vi "CreateQbusListners.vi"(11 "ConnInfo":T1) -> (0 "error out":errorcluster, 3 "Qbus out":refnum<class "Qbus.lvclass">)   [LabVIEW 2017]
uses:
  <vilib>/addons/Qbus/Qbus.lvclass
  <vilib>/addons/InsightCM/Devices/Shared/Common/ServerComm/ServerComm.lvlib
  <vilib>/addons/TimerProcess/TimerProcess.lvlib
  <vilib>/addons/InsightCM/Devices/Shared/Common/DataFlow/test/SpeedBenchmark/Loop1/Loop1.lvlib
  <vilib>/addons/InsightCM/Devices/Shared/Common/DataFlow/test/SpeedBenchmark/Loop2/Loop2.lvlib
  <vilib>/addons/InsightCM/Devices/Shared/Common/DataFlow/test/SpeedBenchmark/Loop3/Loop3.lvlib
  <vilib>/addons/InsightCM/Devices/Shared/Common/DataFlow/test/SpeedBenchmark/Loop4/Loop4.lvlib
  <vilib>/addons/InsightCM/Devices/Shared/Common/DataFlow/test/SpeedBenchmark/Loop5/Loop5.lvlib
  <vilib>/addons/InsightCM/Devices/Shared/Common/DataFlow/test/SpeedBenchmark/Loop6/Loop6.lvlib
  <vilib>/addons/InsightCM/Devices/Shared/Common/DataFlow/test/SpeedBenchmark/Loop7/Loop7.lvlib
  <vilib>/addons/InsightCM/Devices/Shared/Common/DataFlow/test/SpeedBenchmark/Loop8/Loop8.lvlib
  <vilib>/addons/InsightCM/Devices/Shared/Common/DataFlow/test/SpeedBenchmark/Loop9/Loop9.lvlib
  <vilib>/addons/InsightCM/Devices/Shared/Common/DataFlow/test/SpeedBenchmark/Loop10/Loop10.lvlib
  <vilib>/addons/InsightCM/MessageBus/Base/controls/ConnectionInfo.ctl
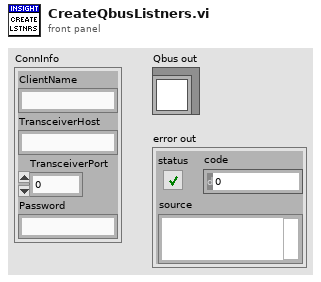
[diagram p1: front panel]
types:
  T1 = typedef "ConnectionInfo.ctl" = cluster{"ClientName":string, "TransceiverHost":string, "TransceiverPort":u16, "Password":string}
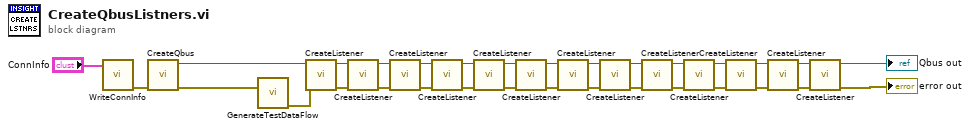
[diagram p0: block diagram]
diagram:
  n1 = call <vilib>:"WriteConnInfo.vi"("connection info"="ConnInfo") -> ("error out"=w12:errorcluster)  [unwired: 10 in]
  n2 = call <vilib>:"CreateQbus.vi"("error in (no error)"=w12) -> ("error out"=w30:errorcluster, "Qbus"=w11:refnum<class "Qbus.lvclass">)  [unwired: 9 in]
  n3 = call <vilib>:"GenerateTestDataFlow.vi"("error in (no error)"=w30) -> ("Error Out"=w20:errorcluster)  [unwired: 10 in]
  n4 = call <vilib>:"CreateListener.vi"("error in (no error)"=w20, "Qbus in"=w11) -> ("error out"=w21:errorcluster, "Qbus out"=w10:refnum<class "Qbus.lvclass">)  [unwired: 8 in]
  n5 = call <vilib>:"CreateListener.vi"("error in (no error)"=w21, "Qbus in"=w10) -> ("error out"=w22:errorcluster, "Qbus out"=w9:refnum<class "Qbus.lvclass">)  [unwired: 8 in]
  n6 = call <vilib>:"CreateListener.vi"("error in (no error)"=w22, "Qbus in"=w9) -> ("error out"=w23:errorcluster, "Qbus out"=w8:refnum<class "Qbus.lvclass">)  [unwired: 8 in]
  n7 = call <vilib>:"CreateListener.vi"("error in (no error)"=w23, "Qbus in"=w8) -> ("error out"=w24:errorcluster, "Qbus out"=w7:refnum<class "Qbus.lvclass">)  [unwired: 8 in]
  n8 = call <vilib>:"CreateListener.vi"("error in (no error)"=w24, "Qbus in"=w7) -> ("error out"=w25:errorcluster, "Qbus out"=w6:refnum<class "Qbus.lvclass">)  [unwired: 8 in]
  n9 = call <vilib>:"CreateListener.vi"("error in (no error)"=w25, "Qbus in"=w6) -> ("error out"=w26:errorcluster, "Qbus out"=w5:refnum<class "Qbus.lvclass">)  [unwired: 8 in]
  n10 = call <vilib>:"CreateListener.vi"("error in (no error)"=w26, "Qbus in"=w5) -> ("error out"=w27:errorcluster, "Qbus out"=w4:refnum<class "Qbus.lvclass">)  [unwired: 8 in]
  n11 = call <vilib>:"CreateListener.vi"("error in (no error)"=w27, "Qbus in"=w4) -> ("error out"=w28:errorcluster, "Qbus out"=w3:refnum<class "Qbus.lvclass">)  [unwired: 8 in]
  n12 = call <vilib>:"CreateListener.vi"("error in (no error)"=w28, "Qbus in"=w3) -> ("error out"=w29:errorcluster, "Qbus out"=w2:refnum<class "Qbus.lvclass">)  [unwired: 8 in]
  n13 = call <vilib>:"CreateListener.vi"("error in (no error)"=w29, "Qbus in"=w2) -> ("error out"=w31:errorcluster, "Qbus out"=w1:refnum<class "Qbus.lvclass">)  [unwired: 8 in]
  n14 = call <vilib>:"CreateListener.vi"("error in (no error)"=w31, "Qbus in"=w1) -> ("error out"=w14:errorcluster, "Qbus out"=w13:refnum<class "Qbus.lvclass">)  [unwired: 8 in]
  n15 = call <vilib>:"CreateListener.vi"("error in (no error)"=w14, "qbus in"=w13) -> ("error out"=w16:errorcluster, "qbus out"=w15:refnum<class "Qbus.lvclass">)  [unwired: 8 in]
  n16 = call <vilib>:"CreateListener.vi"("error in (no error)"=w16, "Qbus in"=w15) -> ("error out"=→"error out":errorcluster, "Qbus out"=→"Qbus out":refnum<class "Qbus.lvclass">)  [unwired: 8 in]
